vi "runBraking.vi"(6 "Fault?":bool, 7 "x acceleration":dbl, 8 "error in (no error)":errorcluster, 9 "Actuators in":T1, 10 "State in":T2, 11 "FullRun in":refnum<class "FullRun.lvclass">) -> (0 "error out":errorcluster, 1 "Actuators out":T1, 2 "State out":T2, 3 "FullRun out":refnum<class "FullRun.lvclass">)   [LabVIEW 2018, in "ControlLibrary.lvlib" / "FullRun.lvclass"]
uses:
  FullRun.lvclass
  TypeDef_ControlState.ctl
  TypeDef_DigitalOuts.ctl
  RunTypeClass/RunType.lvclass
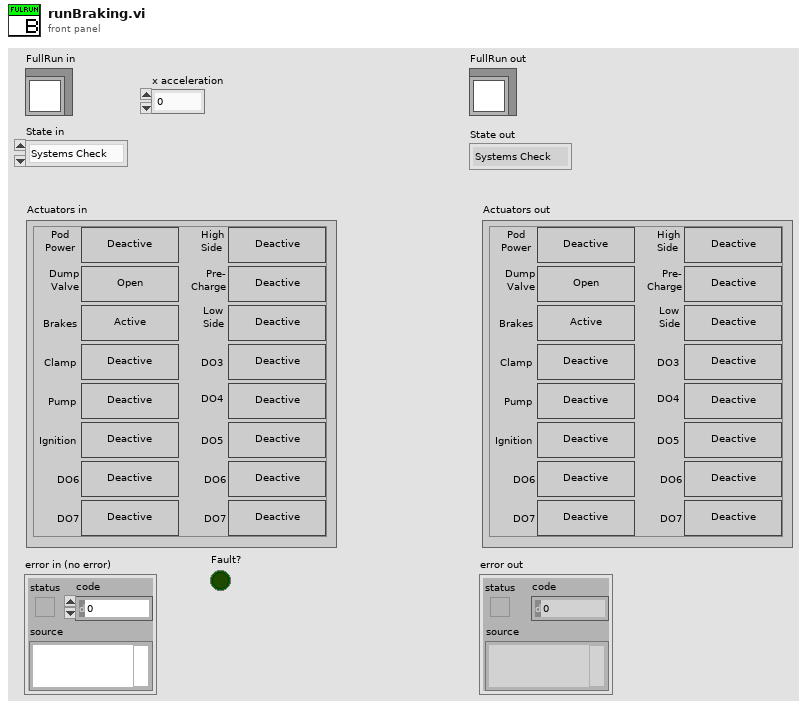
[diagram p1: front panel]
types:
  T1 = typedef "TypeDef_DigitalOuts.ctl" = cluster{"Pod Power":bool, "Dump Valve":bool, "Brakes":bool, "Clamp":bool, "Pump":bool, "Ignition":bool, "DO6":bool, "DO7":bool, "HighSide":bool, "Precharge":bool, "LowSide":bool, "DO3":bool, "DO4":bool, "DO5":bool, "DO62":bool, "DO72":bool}
  T2 = typedef "TypeDef_ControlState.ctl" = enum16{"Systems Check", "Idle", "Ready", "Pushing", "Coast", "Braking", "Fault", "Shutdown", "Service", "Precharge", "Blank"}
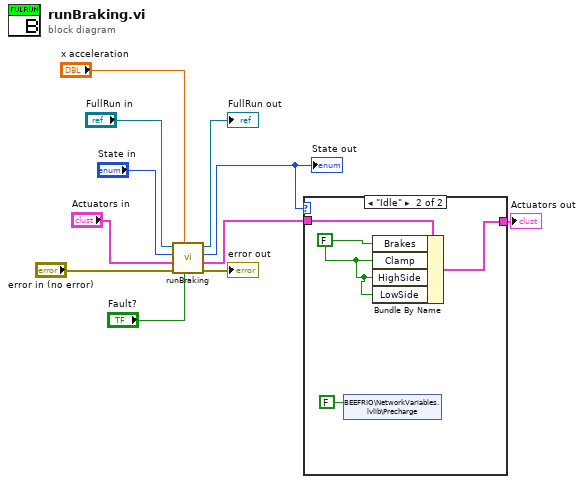
[diagram p0: block diagram]
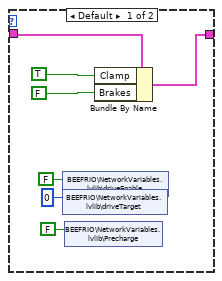
[diagram p2: hidden frame]
diagram:
  n1 = call-parent "runBraking.vi"("Fault?"="Fault?", "x acceleration"="x acceleration", "error in (no error)"="error in (no error)", "Actuators in"="Actuators in", "State in"="State in", "RunType in"="FullRun in") -> ("error out"=→"error out":errorcluster, "Actuators out"=w3:T1, "State out"=w4:T2, "RunType out"=→"FullRun out":refnum<class "FullRun.lvclass">)  [unwired: 2 in]
  "State out" <- w4
  n2 = case shown="\"Idle\"" w4 {
    tunnel: w3 -> [w16 w22]
    tunnel: [w15 w21] -> w2
    frame Default {
      n3 = shared-variable "BEEFRIO\\NetworkVariables.lvlib\\driveEnable"(FALSE ("driveEnable")) -> ()  [unwired: 1 in, 1 out]
      n4 = shared-variable "BEEFRIO\\NetworkVariables.lvlib\\driveTarget"(i16 0 ("driveTarget")) -> ()  [unwired: 1 in, 1 out]
      n5 = shared-variable "BEEFRIO\\NetworkVariables.lvlib\\Precharge"(FALSE ("Precharge")) -> ()  [unwired: 1 in, 1 out]
      n6 = Bundle By Name(cluster=w16, "Clamp"=TRUE ("Actuators.Clamp"), "Brakes"=FALSE ("Actuators.Brakes")) -> (w15:T1)
    }
    frame "Idle" {
      w19 = FALSE ("Actuators.Brakes")
      n7 = shared-variable "BEEFRIO\\NetworkVariables.lvlib\\Precharge"(FALSE ("Precharge")) -> ()  [unwired: 1 in, 1 out]
      n8 = Bundle By Name(cluster=w22, "Brakes"=w19, "Clamp"=w19, "HighSide"=w19, "LowSide"=w19) -> (w21:T1)
    }
  }
  "Actuators out" <- w2
